vi "Disconnect.vi"(6 "Hold":bool, 8 "error in":errorcluster) -> (0 "error out":errorcluster)   [LabVIEW 2014, in "TCP.lvlib"]
uses:
  TCP.lvlib
  support/Message Queue/Message Queue.lvlib
  support/Message Queue/Enqueue Message (Single).vi
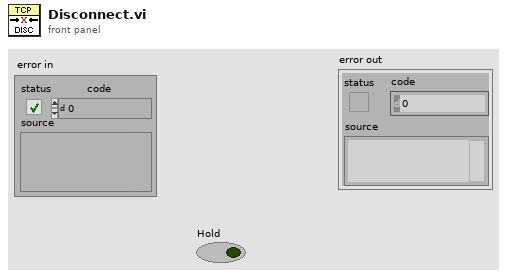
[diagram p1: front panel]
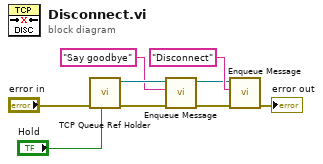
[diagram p0: block diagram]
diagram:
  n1 = call "TCP Queue Ref Holder.vi"("Hold"="Hold", "error in (no error)"="error in") -> ("error out"=w5:errorcluster, "Input Queue"=w3:refnum<queue>)  [unwired: 8 in]
  n2 = call-poly "Enqueue Message.vi"("error in (no error)"=w5, "Message"="Say goodbye", "Message Queue"=w3) -> ("error out"=w4:errorcluster, "dup Message Queue"=w2:refnum<queue>)  [unwired: 7 in]
  n3 = call-poly "Enqueue Message.vi"("error in (no error)"=w4, "Message"="Disconnect", "Message Queue"=w2) -> ("error out"=→"error out":errorcluster)  [unwired: 7 in, 1 out]
